vi "writeNewScripts.vi"(8 "error in (no error)":errorcluster, 10 "delayAll":bool, 11 "ScanCreator in":refnum<class "ScanCreator.lvclass">) -> (0 "error out":errorcluster, 1 "Values":string[](array[string]), 2 "scriptListArray":refnum<class "ScriptEventList.lvclass">[](array[class]), 3 "ScanCreator out":refnum<class "ScanCreator.lvclass">, 4 "scanType":string)   [LabVIEW 2011, in "Views.lvlib" / "ScriptEditor.lvlib" / "ScanCreator.lvclass"]
uses:
  ScanCreator.lvclass
  Tools/Scripting/ScriptingEvent/ScriptEventList/ScriptEventList.lvclass
  ScanCreator.lvclass/ScanCreator.ctl
  Tools/Scripting/ScriptingEvent/ScriptEvent.lvclass
  Tools/Scripting/ScriptingEvent/ScriptEvents/Delay/Delay.lvclass
  Tools/Scripting/ScriptingEvent/ScriptEvents/Ramp/RampEvent/RampEvent.lvclass
  Tools/Scripting/ScriptingEvent/ScriptEvents/Rf Event/rf.lvclass
  Tools/DatabaseHelpers/Database Objects/Channel/Channel.lvclass
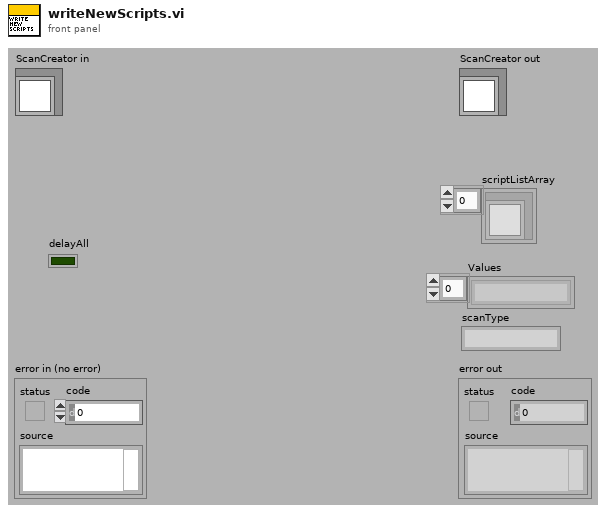
[diagram p1: front panel]
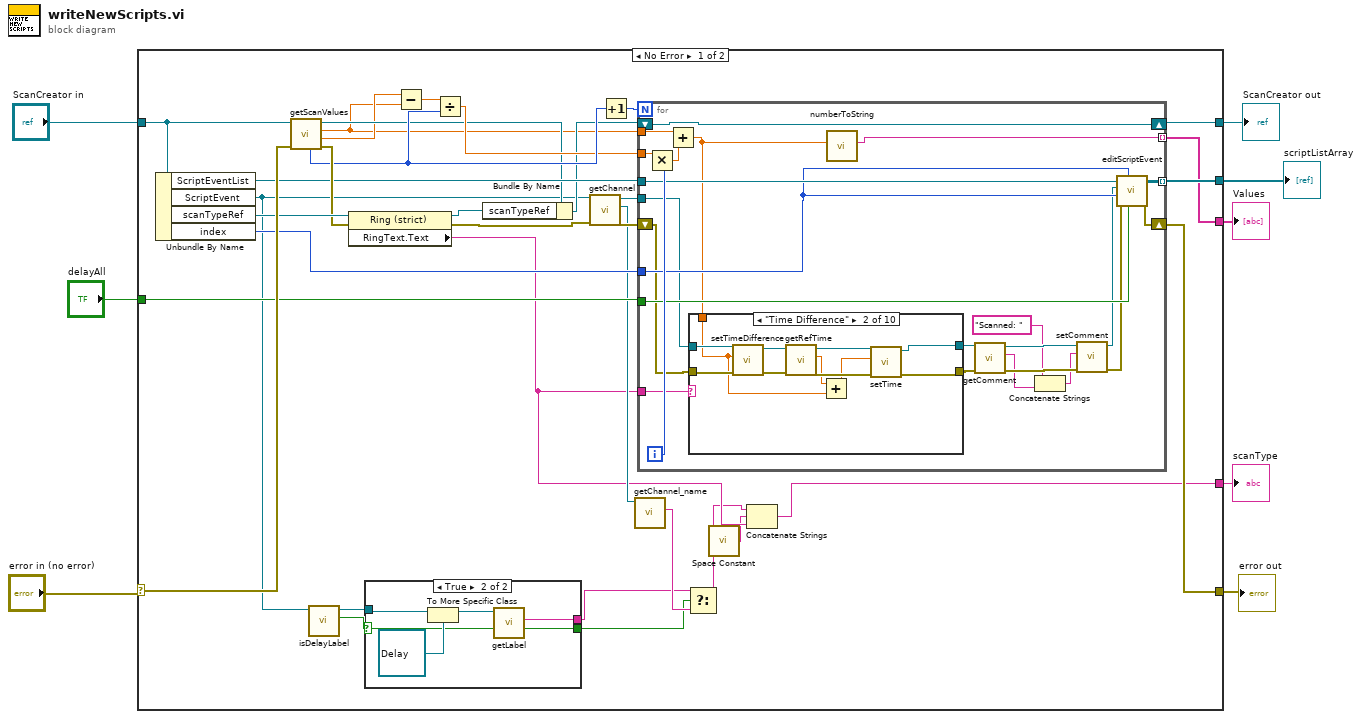
[diagram p0: block diagram]
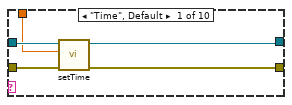
[diagram p3: hidden frame]
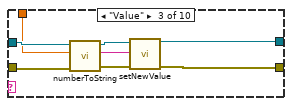
[diagram p4: hidden frame]
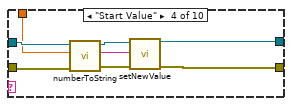
[diagram p5: hidden frame]
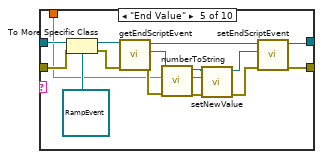
[diagram p6: hidden frame]
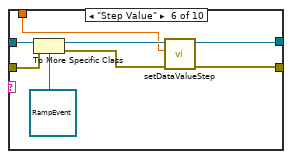
[diagram p7: hidden frame]
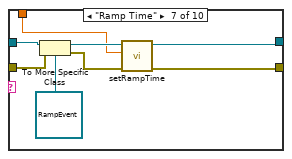
[diagram p8: hidden frame]
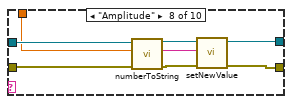
[diagram p9: hidden frame]
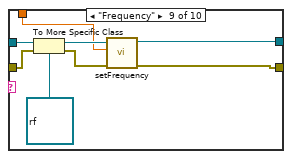
[diagram p10: hidden frame]
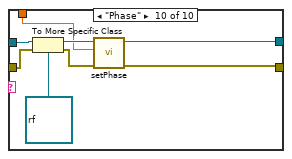
[diagram p11: hidden frame]
diagram:
  n1 = case shown="No Error" "error in (no error)" {
    selector: "error in (no error)" -> [w41 w162]
    tunnel: [w27 w162] -> w7
    tunnel: [w31 w161] -> w5
    tunnel: "ScanCreator in" -> [w42 w161]
    tunnel: "delayAll" -> [w33 _]
    tunnel: [w32 _] -> w3
    tunnel: [w25 _] -> w2
    tunnel: [w17 _] -> w1
    frame No Error {
      n2 = Unbundle By Name(w42) -> ("ScriptEventList"=w38:refnum<class "ScriptEventList.lvclass">, "ScriptEvent"=w15:refnum<class "ScriptEvent.lvclass">, "scanTypeRef"=w40:refnum<vi>, "index"=w34:i16)
      n3 = call "getScanValues.vi"("error in (no error)"=w41, "ScanCreator in"=w42) -> ("error out"=w39:errorcluster, "stop"=w24:dbl, "start"=w23:dbl, "ScanCreator out"=w30:refnum<class "ScanCreator.lvclass">, "step"=w36:i16)  [unwired: 4 in, 1 out]
      n4 = call "isDelayLabel.vi"("ScriptEvent in"=w15) -> ("delay"=w14:bool, "ScriptEvent out"=w13:refnum<class "ScriptEvent.lvclass">)  [unwired: 8 in, 1 out]
      n5 = property class="Ring (strict)"(reference=w40, error in=w39) -> (reference out=w28:refnum<vi>, error out=w21:errorcluster, "RingText.Text"=w18:string)
      n6 = case shown="True" w14 {
        selector: w14 -> [w43 w44]
        tunnel: w13 -> [_ w48]
        tunnel: [_ w45] -> w10
        tunnel: [w43 w44] -> w11
        frame False {
        }
        frame True {
          n7 = To More Specific Class(target class=refnum<class "Delay.lvclass"> refnum ("Tools.lvlib:Scripting.lvlib:Delay.lvclass"), reference=w48) -> (specific class reference=w46:refnum<class "Delay.lvclass">)  [unwired: 1 in, 1 out]
          n8 = call "getLabel.vi"("Delay in"=w46) -> ("label"=w45:string)  [unwired: 8 in, 2 out]
        }
      }
      n9 = Subtract(x=w24, y=w23) -> (x-y=w37:dbl)
      n10 = Divide(x=w37, y=w36) -> (x/y=w35:dbl)
      n11 = Bundle By Name(cluster=w30, "scanTypeRef"=w28) -> (w29:refnum<class "ScanCreator.lvclass">)
      n12 = call-dynamic "getChannel.vi"("error in (no error)"=w21, "ScriptEvent.lvclass in"=w15) -> ("error out"=w22:errorcluster, "Channel.lvclass"=w19:refnum<class "Channel.lvclass">, "ScriptEvent.lvclass out"=w20:refnum<class "ScriptEvent.lvclass">)  [unwired: 7 in]
      n13 = Increment(x=w36) -> (x+1=w26:i16)
      n14 = call "getChannel_name.vi"("Channel.lvclass in"=w19) -> ("channel_name"=w12:string)  [unwired: 8 in, 2 out]
      n15 = for {
        N: w26 -> [_]
        tunnel: w35 -> [w71]
        tunnel: w20 -> [w62]
        tunnel: w23 -> [w72]
        tunnel: w38 -> [w68]
        tunnel: w34 -> [w67]
        tunnel: w33 -> [w66]
        tunnel: [w65] -> w32 mode=indexing
        shift-right: [w64] -> w27
        shift-left: w22 -> [w61]
        shift-right: [w63] -> w31
        shift-left: w29 -> [w63]
        tunnel: w18 -> [w60]
        tunnel: [w58] -> w25 mode=indexing
        i -> [w70]
        n16 = Multiply(x=w71, y=w70) -> (x*y=w69:dbl)
        n17 = Add(x=w72, y=w69) -> (x+y=w59:dbl)
        n18 = case shown="\"Time Difference\"" w60 {
          tunnel: w62 -> [w77 w88 w90 w98 w120 w127 w135 w144 w152 w159]
          tunnel: w61 -> [w74 w87 w91 w99 w118 w126 w134 w138 w151 w158]
          tunnel: [w75 w78 w95 w103 w109 w123 w129 w141 w145 w153] -> w56
          tunnel: [w76 w79 w96 w104 w107 w124 w130 w142 w146 w154] -> w57
          tunnel: w59 -> [w73 w81 w89 w97 w113 w122 w131 w137 w147 w155]
          frame "Time", Default {
            n19 = call "setTime.vi"("error in (no error)"=w74, "time"=w73, "ScriptEvent.lvclass in"=w77) -> ("error out"=w75:errorcluster, "ScriptEvent.lvclass out"=w76:refnum<class "ScriptEvent.lvclass">)  [unwired: 7 in]
          }
          frame "Time Difference" {
            n20 = call "setTimeDifference.vi"("error in (no error)"=w87, "time difference"=w81, "ScriptEvent.lvclass in"=w88) -> ("error out"=w85:errorcluster, "ScriptEvent.lvclass out"=w86:refnum<class "ScriptEvent.lvclass">)  [unwired: 7 in]
            n21 = call "getRefTime.vi"("error in (no error)"=w85, "ScriptEvent.lvclass in"=w86) -> ("error out"=w83:errorcluster, "refTime"=w82:dbl, "ScriptEvent.lvclass out"=w84:refnum<class "ScriptEvent.lvclass">)  [unwired: 7 in]
            n22 = Add(x=w82, y=w81) -> (x+y=w80:dbl)
            n23 = call "setTime.vi"("error in (no error)"=w83, "time"=w80, "ScriptEvent.lvclass in"=w84) -> ("error out"=w78:errorcluster, "ScriptEvent.lvclass out"=w79:refnum<class "ScriptEvent.lvclass">)  [unwired: 7 in]
          }
          frame "Value" {
            n24 = call "numberToString.vi"("error in (no error)"=w91, "Numeric"=w89, "ScriptEvent in"=w90) -> ("error out"=w92:errorcluster, "String"=w93:string, "ScriptEvent out"=w94:refnum<class "ScriptEvent.lvclass">)  [unwired: 6 in]
            n25 = call "setNewValue.vi"("error in (no error)"=w92, "newValue"=w93, "ScriptEvent.lvclass in"=w94) -> ("error out"=w95:errorcluster, "ScriptEvent.lvclass out"=w96:refnum<class "ScriptEvent.lvclass">)  [unwired: 7 in]
          }
          frame "Start Value" {
            n26 = call "numberToString.vi"("error in (no error)"=w99, "Numeric"=w97, "ScriptEvent in"=w98) -> ("error out"=w100:errorcluster, "String"=w101:string, "ScriptEvent out"=w102:refnum<class "ScriptEvent.lvclass">)  [unwired: 6 in]
            n27 = call "setNewValue.vi"("error in (no error)"=w100, "newValue"=w101, "ScriptEvent.lvclass in"=w102) -> ("error out"=w103:errorcluster, "ScriptEvent.lvclass out"=w104:refnum<class "ScriptEvent.lvclass">)  [unwired: 7 in]
          }
          frame "End Value" {
            n28 = To More Specific Class(target class=refnum<class "RampEvent.lvclass"> refnum ("Tools.lvlib:Scripting.lvlib:RampEvent.lvclass"), reference=w120, error in=w118) -> (specific class reference=w117:refnum<class "RampEvent.lvclass">, error out=w116:errorcluster)
            n29 = call "getEndScriptEvent.vi"("error in (no error)"=w116, "RampEvent.lvclass in"=w117) -> ("error out"=w114:errorcluster, "ScriptEvent.lvclass"=w115:refnum<class "ScriptEvent.lvclass">, "RampEvent.lvclass out"=w108:refnum<class "RampEvent.lvclass">)  [unwired: 7 in]
            n30 = call "numberToString.vi"("error in (no error)"=w114, "Numeric"=w113, "ScriptEvent in"=w115) -> ("error out"=w111:errorcluster, "String"=w110:string, "ScriptEvent out"=w112:refnum<class "ScriptEvent.lvclass">)  [unwired: 6 in]
            n31 = call "setNewValue.vi"("error in (no error)"=w111, "newValue"=w110, "ScriptEvent.lvclass in"=w112) -> ("error out"=w106:errorcluster, "ScriptEvent.lvclass out"=w105:refnum<class "ScriptEvent.lvclass">)  [unwired: 7 in]
            n32 = call "setEndScriptEvent.vi"("error in (no error)"=w106, "endScriptEvent.lvclass"=w105, "RampEvent.lvclass in"=w108) -> ("error out"=w109:errorcluster, "RampEvent.lvclass out"=w107:refnum<class "RampEvent.lvclass">)  [unwired: 7 in]
          }
          frame "Step Value" {
            n33 = To More Specific Class(target class=refnum<class "RampEvent.lvclass"> refnum ("Tools.lvlib:Scripting.lvlib:RampEvent.lvclass"), reference=w127, error in=w126) -> (specific class reference=w125:refnum<class "RampEvent.lvclass">, error out=w121:errorcluster)
            n34 = call "setDataValueStep.vi"("error in (no error)"=w121, "dataValueStep"=w122, "RampEvent.lvclass in"=w125) -> ("error out"=w123:errorcluster, "RampEvent.lvclass out"=w124:refnum<class "RampEvent.lvclass">)  [unwired: 7 in]
          }
          frame "Ramp Time" {
            n35 = To More Specific Class(target class=refnum<class "RampEvent.lvclass"> refnum ("Tools.lvlib:Scripting.lvlib:RampEvent.lvclass"), reference=w135, error in=w134) -> (specific class reference=w133:refnum<class "RampEvent.lvclass">, error out=w132:errorcluster)
            n36 = call "setRampTime.vi"("error in (no error)"=w132, "rampTime"=w131, "RampEvent.lvclass in"=w133) -> ("error out"=w129:errorcluster, "RampEvent.lvclass out"=w130:refnum<class "RampEvent.lvclass">)  [unwired: 7 in]
          }
          frame "Amplitude" {
            n37 = call "numberToString.vi"("error in (no error)"=w138, "Numeric"=w137, "ScriptEvent in"=w144) -> ("error out"=w140:errorcluster, "String"=w139:string, "ScriptEvent out"=w143:refnum<class "ScriptEvent.lvclass">)  [unwired: 6 in]
            n38 = call "setNewValue.vi"("error in (no error)"=w140, "newValue"=w139, "ScriptEvent.lvclass in"=w143) -> ("error out"=w141:errorcluster, "ScriptEvent.lvclass out"=w142:refnum<class "ScriptEvent.lvclass">)  [unwired: 7 in]
          }
          frame "Frequency" {
            n39 = To More Specific Class(target class=refnum<class "rf.lvclass"> refnum ("Tools.lvlib:Scripting.lvlib:rf.lvclass"), reference=w152, error in=w151) -> (specific class reference=w149:refnum<class "rf.lvclass">, error out=w148:errorcluster)
            n40 = call "setFrequency.vi"("error in (no error)"=w148, "frequency"=w147, "rf in"=w149) -> ("error out"=w145:errorcluster, "rf out"=w146:refnum<class "rf.lvclass">)  [unwired: 7 in]
          }
          frame "Phase" {
            n41 = To More Specific Class(target class=refnum<class "rf.lvclass"> refnum ("Tools.lvlib:Scripting.lvlib:rf.lvclass"), reference=w159, error in=w158) -> (specific class reference=w157:refnum<class "rf.lvclass">, error out=w156:errorcluster)
            n42 = call "setPhase.vi"("error in (no error)"=w156, "phase"=w155, "rf in"=w157) -> ("error out"=w153:errorcluster, "rf out"=w154:refnum<class "rf.lvclass">)  [unwired: 7 in]
          }
        }
        n43 = call "numberToString.vi"("Numeric"=w59) -> ("String"=w58:string)  [unwired: 8 in, 2 out]
        n44 = call "getComment.vi"("error in (no error)"=w56, "ScriptEvent.lvclass in"=w57) -> ("error out"=w54:errorcluster, "comment"=w53:string, "ScriptEvent.lvclass out"=w55:refnum<class "ScriptEvent.lvclass">)  [unwired: 7 in]
        n45 = Concatenate Strings("Scanned: ", w53) -> (w51:string)
        n46 = call-dynamic "setComment.vi"("error in (no error)"=w54, "comment"=w51, "ScriptEvent.lvclass in"=w55) -> ("error out"=w49:errorcluster, "ScriptEvent.lvclass out"=w50:refnum<class "ScriptEvent.lvclass">)  [unwired: 7 in]
        n47 = call "editScriptEvent.vi"("delayAll"=w66, "selectedIndex"=w67, "error in (no error)"=w49, "index"=w67, "ScriptEvent"=w50, "ScriptEventList in"=w68) -> ("error out"=w64:errorcluster, "ScriptEventList out"=w65:refnum<class "ScriptEventList.lvclass">)  [unwired: 4 in]
      }
      n48 = Select(t=w10, s=w11, f=w12) -> (s? t:f=w9:string)
      n49 = call <vilib>:"Space Constant.vi"() -> ("String"=w16:string)
      n50 = Concatenate Strings(w9, w16, w18) -> (w17:string)
    }
    frame Error {
    }
  }
  "error out" <- w7
  "ScanCreator out" <- w5
  "scriptListArray" <- w3
  "Values" <- w2
  "scanType" <- w1
